vi "post_dcs_points.vi"(8 "error in (no error)":errorcluster, 11 "DCS points":T1={"Integer Timestamp"=8, "X"=2.0, "Y"=3.0, "DCS spot ID"=0}) -> (0 "error out":errorcluster)   [LabVIEW 2013]
doc: "Adds a new row to the dcs_points table."
uses:
  User Interface/Controls/dcs points.ctl
  <vilib>/addons/database/NI_Database_API.lvlib
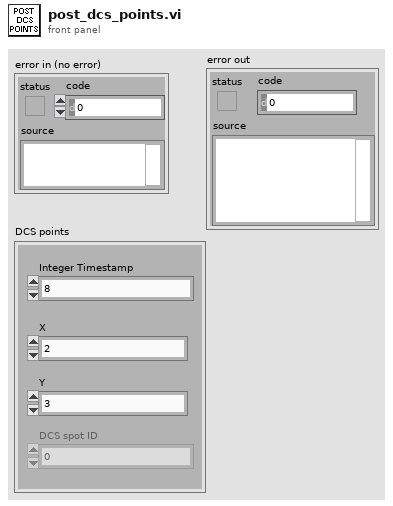
[diagram p1: front panel]
types:
  T1 = typedef "dcs points.ctl" = cluster{"Integer Timestamp":i64, "X":dbl, "Y":dbl, "DCS spot ID":i32}
  T2 = typedef "NI_Database_API.lvlib/Conn ObjectReference.ctl" = refnum<k1>
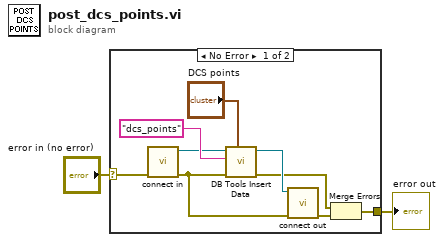
[diagram p0: block diagram]
diagram:
  n1 = case shown="No Error" "error in (no error)" {
    selector: "error in (no error)" -> [w11 w12]
    tunnel: [w3 w12] -> w1
    frame No Error {
      n2 = call "connect in.vi"("error in (no error)"=w11) -> ("error out"=w5:errorcluster, "Database Connection"=w9:T2)  [unwired: 7 in]
      n3 = call <vilib>:"DB Tools Insert Data.vi"("data"="DCS points", "error in (no error)"=w5, "table"="dcs_points", "connection reference"=w9) -> ("error out"=w6:errorcluster, "connection reference out"=w8:T2)  [unwired: 6 in]
      n4 = call "connect out.vi"("error in (no error)"=w5, "connection reference"=w8) -> ("error out"=w4:errorcluster)  [unwired: 9 in]
      n5 = Merge Errors(w6, w4) -> (w3:errorcluster)
    }
    frame Error {
    }
  }
  "error out" <- w1
